vi "LVClass_WavefrontCorrectorSet get plane commands.vi"(0 "WavefrontCorrectorSet in":refnum<class "WavefrontCorrectorSet.lvclass">, 11 "error in (no error)":errorcluster) -> (4 "WavefrontCorrectorSet out":refnum<class "WavefrontCorrectorSet.lvclass">, 6 "PlaneCommand_1D":sgl[](array[numeric]), 15 "error out":errorcluster)   [LabVIEW 2020, in "WavefrontCorrectorSet.lvclass"]
doc: "WavefrontCorrector commands to flat mirror shape getter.\n\n--------------------------------------------------------------------------------\n\n<B>wavefrontcorrector_setIn </B> : WavefrontCorrectorSet object.\n<B>wavefrontcorrector_setOut </B> : WavefrontCorrectorSet object.\n<B>flat_command </B> : Array of commands to apply to have a flat wavefront corrector surface.\n<B>ErrorIn </B> : Error\n<B>ErrorOut </B> : Error\n\n--------------------------------------------------------------------------------"
uses:
  WavefrontCorrectorSet.lvclass
  WavefrontCorrectorSet.lvclass/WavefrontCorrectorSet.ctl
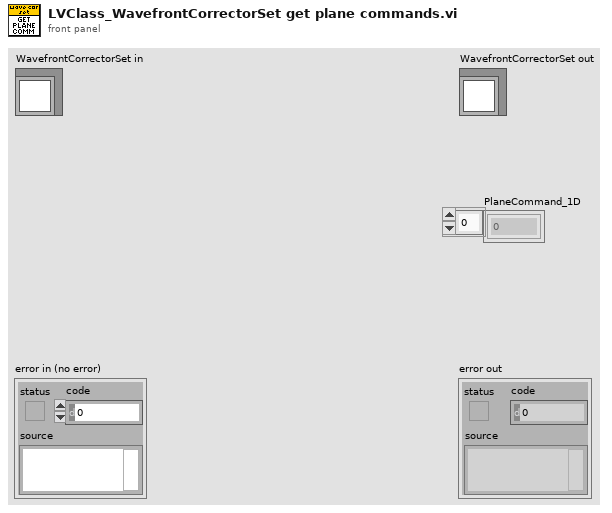
[diagram p1: front panel]
types:
  T1 = typedef "ClassID.ctl" = i64
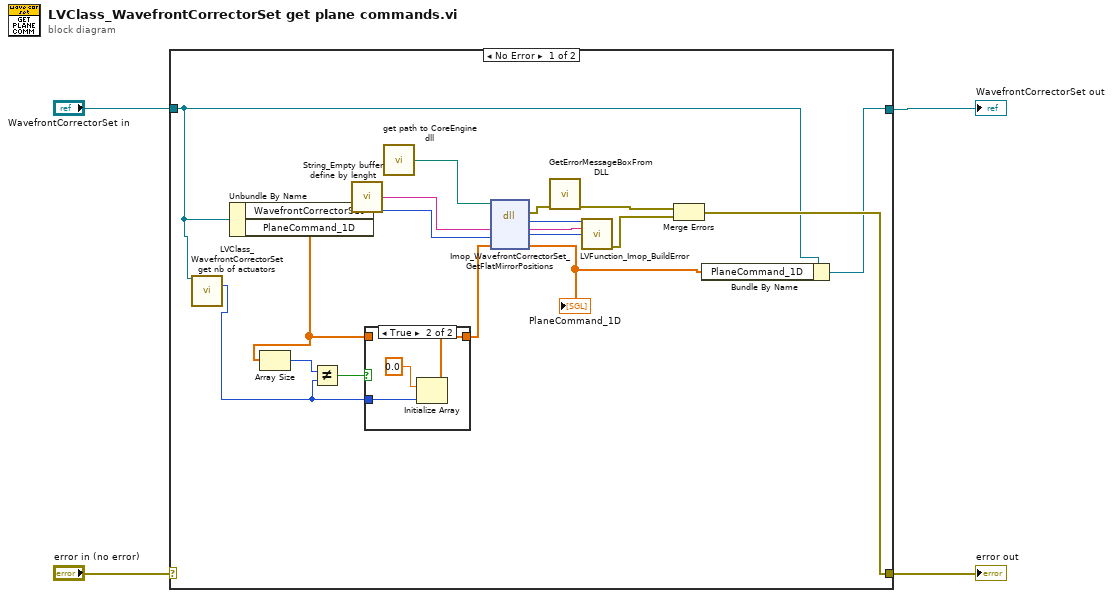
[diagram p0: block diagram]
diagram:
  n1 = case shown="No Error" "error in (no error)" {
    selector: "error in (no error)" -> [_ w28]
    tunnel: [w15 w28] -> w2
    tunnel: [w7 w27] -> w1
    tunnel: "WavefrontCorrectorSet in" -> [w8 w27]
    frame No Error {
      n2 = call "LVClass_WavefrontCorrectorSet get nb of actuators.vi"("WavefrontCorrectorSet in"=w8) -> ("ActuatorsNumber"=w6:i32)  [unwired: 12 in, 2 out]
      n3 = Unbundle By Name(w8) -> ("WavefrontCorrectorSet"=w14:T1, "PlaneCommand_1D"=w11:sgl[])
      n4 = Array Size(array=w11) -> (size(s)=w12:i32)
      n5 = Not Equal?(x=w12, y=w6) -> (x != y?=w13:bool)
      n6 = call "String_Empty buffer define by lenght.vi"() -> ("Empty buffer"=w20:string)  [unwired: 1 in]
      n7 = case shown="True" w13 {
        tunnel: [w23 w25] -> w10
        tunnel: w6 -> [_ w26]
        tunnel: w11 -> [w23 _]
        frame False {
        }
        frame True {
          n8 = Initialize Array(sgl 0.0 ("PlaneCommand_1D"), w26) -> (w25:sgl[])
        }
      }
      n9 = call "get path to CoreEngine dll.vi"() -> ("path to wavekit library"=w19:path)  [unwired: 14 in, 1 out]
      n10 = dll-call lib="D:/soft/HASO_v3/SVN_trunk/ImOpCoreEngine4_LV2011/DLLs/c_interface_vc100.dll" fn="Imop_WavefrontCorrectorSet_GetFlatMirrorPositions"(path in=w19, "message"=w20, "WavefrontCorrectionSet"=w14, "PlaneCommand_1D"=w10) -> (error out=w18:errorcluster, "return type"=w22:i32, "message"=w21:string, "WavefrontCorrectionSet"=w5:i64, "PlaneCommand_1D"=w9:sgl[])  [unwired: 2 in, 1 out]
      "PlaneCommand_1D" <- w9
      n11 = call "GetErrorMessageBoxFromDLL.vi"("error IN"=w18) -> ("error OUT"=w17:errorcluster)  [unwired: 10 in]
      n12 = call "LVFunction_Imop_BuildError.vi"("code"=w22, "String to Prepend to source (\"\")"=w21, "Adresse"=w5) -> ("error out"=w16:errorcluster)  [unwired: 12 in]
      n13 = Merge Errors(w17, w16) -> (w15:errorcluster)
      n14 = Bundle By Name(cluster=w8, "PlaneCommand_1D"=w9) -> (w7:refnum<class "WavefrontCorrectorSet.lvclass">)
    }
    frame Error {
    }
  }
  "error out" <- w2
  "WavefrontCorrectorSet out" <- w1
